vi "json test.vi"(11 "Parameters Enum":T3) -> ()   [LabVIEW 2020]
uses:
  Sensor General Class/Parameters Enum.ctl
  Sensor General Class/Sensor General Class.lvclass
panel:
  out "output cluster":T1
  in  "Configuration 2":T2(array[cluster])
  out "JSON string":string
  out "Configuration":T2(array[cluster])
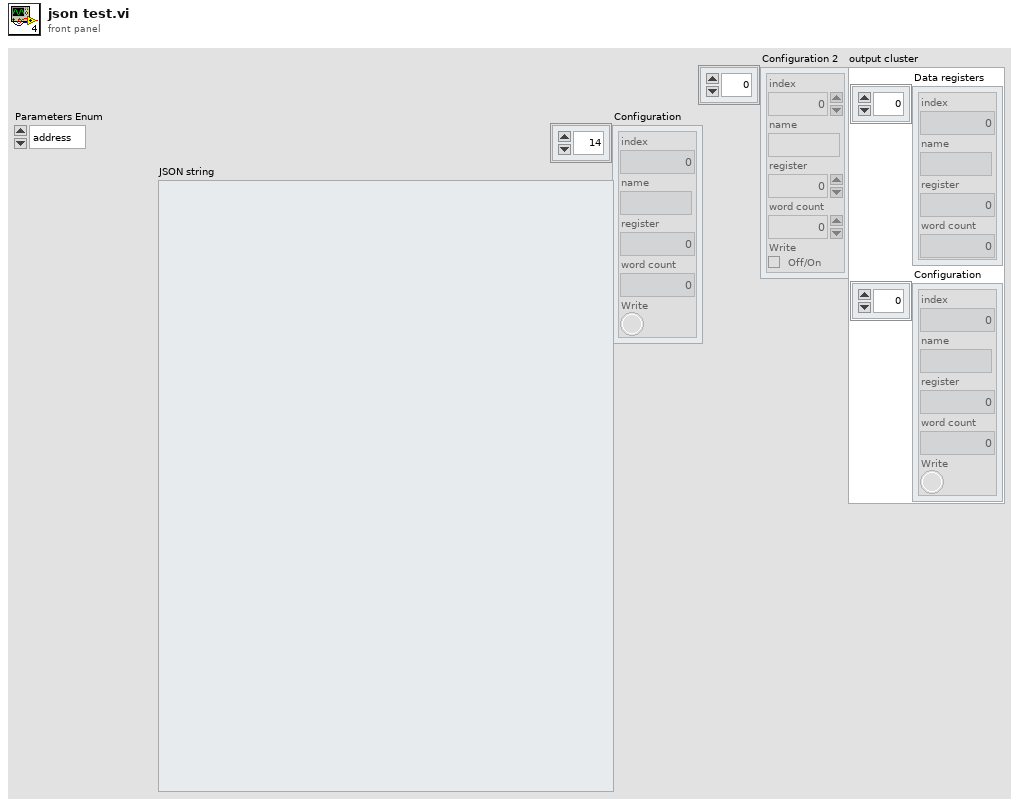
[diagram p1: front panel]
types:
  T1 = cluster{"Data registers":cluster{"index":i32, "name":string, "register":u16, "word count":u16}[], "Configuration":cluster{"index":i32, "name":string, "register":u16, "word count":u16, "Write":bool}[]}
  T2 = cluster{"index":i32, "name":string, "register":u16, "word count":u16, "Write":bool}[]
  T3 = typedef "Sensor General Class.lvclass/Parameters Enum.ctl" = enum16{"address", "baud rate", "parity check", "load", "insulating gas", "additional component", "s/n", "hardware version", "firmware version", "humidity enable", "tag", "pressure offset", "humidity offset", "temperature offset", "service code"}
  T4 = cluster{"index":i32, "name":string, "register":u16, "word count":u16}[]
  T5 = cluster{"index":i32, "name":string, "register":u16, "word count":u16, "Write":bool}
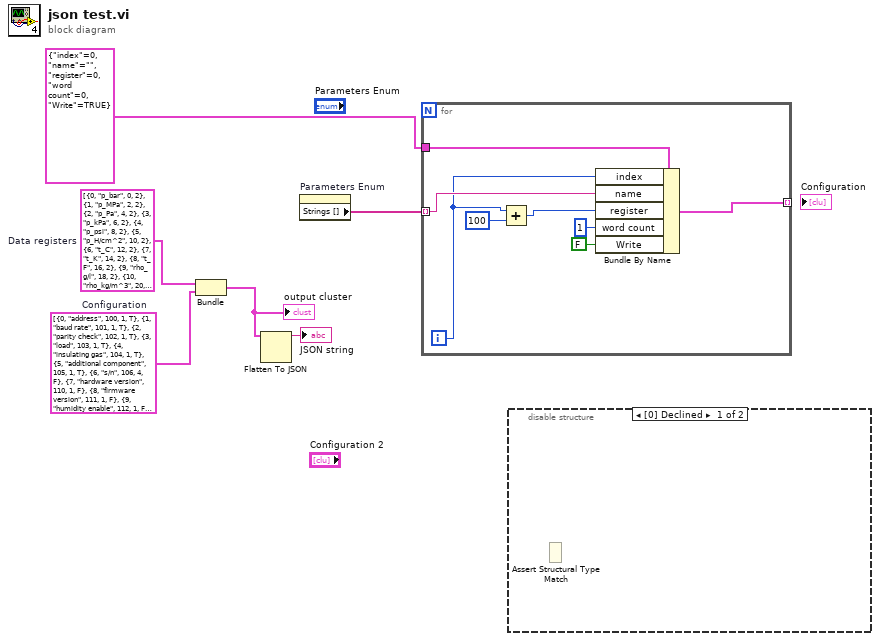
[diagram p0: block diagram]
diagram:
  w4 = T4 [{"index"=0, "name"="p_bar", "register"=0, "word count"=2}, {"index"=1, "name"="p_MPa", "register"=2, "word count"=2}, {"index"=2, "name"="p_Pa", "register"=4, "word count"=2}, {"index"=3, "name"="p_kPa", "register"=6, "word count"=2}, {"index"=4, "name"="p_psi", "register"=8, "word count"=2}, {"index"=5, "name"="p_H/cm^2", "register"=10, "word count"=2}, {"index"=6, "name"="t_C", "register"=12, "word count"=2}, {"index"=7, "name"="t_K", "register"=14, "word count"=2}, {"index"=8, "name"="t_F", "register"=16, "word count"=2}, {"index"=9, "name"="rho_g/l", "register"=18, "word count"=2}, {"index"=10, "name"="rho_kg/m^3", "register"=20, "word count"=2}, {"index"=11, "name"="p20_bar", "register"=22, "word count"=2}, {"index"=12, "name"="related p20_bar", "register"=58, "word count"=2}, {"index"=13, "name"="p20_MPa", "register"=60, "word count"=2}, {"index"=14, "name"="related p20_MPa", "register"=62, "word count"=2}, {"index"=15, "name"="Tf_SF6", "register"=24, "word count"=2}, {"index"=16, "name"="Td_sf6", "register"=26, "word count"=2}, {"index"=17, "name"="tank Tf_SF6", "register"=28, "word count"=2}, {"index"=18, "name"="tank Td_SF6", "register"=30, "word count"=2}, {"index"=19, "name"="Tf_N2", "register"=32, "word count"=2}, {"index"=20, "name"="Td_N2", "register"=34, "word count"=2}, {"index"=21, "name"="tank Tf_N2", "register"=36, "word count"=2}, {"index"=22, "name"="tank Td_N2", "register"=38, "word count"=2}, {"index"=23, "name"="ppm_v SF6", "register"=40, "word count"=2}, {"index"=24, "name"="ppm_w SF6", "register"=42, "word count"=2}, {"index"=25, "name"="ppm_v N2", "register"=44, "word count"=2}, {"index"=26, "name"="ppm_w N2", "register"=46, "word count"=2}, {"index"=27, "name"="rH", "register"=48, "word count"=2}]  # Data registers
  w3 = T2 [{"index"=0, "name"="address", "register"=100, "word count"=1, "Write"=TRUE}, {"index"=1, "name"="baud rate", "register"=101, "word count"=1, "Write"=TRUE}, {"index"=2, "name"="parity check", "register"=102, "word count"=1, "Write"=TRUE}, {"index"=3, "name"="load", "register"=103, "word count"=1, "Write"=TRUE}, {"index"=4, "name"="insulating gas", "register"=104, "word count"=1, "Write"=TRUE}, {"index"=5, "name"="additional component", "register"=105, "word count"=1, "Write"=TRUE}, {"index"=6, "name"="s/n", "register"=106, "word count"=4, "Write"=FALSE}, {"index"=7, "name"="hardware version", "register"=110, "word count"=1, "Write"=FALSE}, {"index"=8, "name"="firmware version", "register"=111, "word count"=1, "Write"=FALSE}, {"index"=9, "name"="humidity enable", "register"=112, "word count"=1, "Write"=FALSE}, {"index"=10, "name"="tag", "register"=113, "word count"=16, "Write"=FALSE}, {"index"=11, "name"="pressure offset", "register"=140, "word count"=1, "Write"=TRUE}, {"index"=12, "name"="humidity offset", "register"=139, "word count"=1, "Write"=TRUE}, {"index"=13, "name"="temperature offset", "register"=138, "word count"=1, "Write"=TRUE}, {"index"=14, "name"="service code", "register"=800, "word count"=1, "Write"=TRUE}]  # Configuration
  n1 = Bundle("Data registers"=w4, "Configuration"=w3) -> (w2:T1)  [unwired: 1 in]
  "output cluster" <- w2
  n2 = Flatten To JSON(anything=w2) -> (JSON string=→"JSON string":string)  [unwired: 2 in, 1 out]
  n3 = property on="Parameters Enum" class="Enum (strict)"() -> ("Strings []"=w6:string[])  [unwired: 2 in, 2 out]
  n4 = for {
    tunnel: w6 -> [w13] mode=indexing
    tunnel: T5 {"index"=0, "name"="", "register"=0, "word count"=0, "Write"=TRUE} ("Cluster 2") -> [w14]
    tunnel: [w8] -> _ mode=indexing
    i -> [w12]
    n5 = Add(x=w12, y=100) -> (x+y=w10:i32)
    n6 = Bundle By Name(cluster=w14, "index"=w12, "name"=w13, "register"=w10, "word count"=u16 1, "Write"=FALSE) -> (w8:T5)
  }
  n7 = disable-structure shown="[0] Declined" {
    frame Disabled {
      n8 = Assert Structural Type Match() -> ()  [unwired: 2 in]
    }
    frame Enabled {
    }
  }
